vi "Trabalho2.vi"() -> ()   [LabVIEW 2009]
uses:
  <vilib>/NXT/Block Support/NXT_InputPort.ctl
  <vilib>/NXT/Block Support/NXT_ButtonSelector.ctl
  <vilib>/NXT/Subs/MotorOutput.ctl
  <vilib>/NXT/Dual Mode Library/Waits/Wait_Num.vi
  <vilib>/NXT/Dual Mode Library/Display/drawText.vi
  <vilib>/NXT/Dual Mode Library/Sensors/Light_On.vi
  <vilib>/NXT/Dual Mode Library/Sensors/readNXTButton.vi
  <vilib>/NXT/Dual Mode Library/Sensors/Touch_Pressed.vi
  <vilib>/NXT/Dual Mode Library/Sensors/Sound_dB.vi
  <vilib>/NXT/Dual Mode Library/Sensors/Sonar_cm.vi
  <vilib>/NXT/Subs/NXT_SteeringOutputPort.ctl
panel:
  out "Verificacao":bool[](array[boolean])
  out "Cor Inicial":i16
  out "Toque\nPressionado":bool
  out "Visor":string
  out "Ruído":i16(slide) scale=0.0..100.0
  out "Luminosidade":i16
  out "Distância":i16
  out "Botao\nPressionado":bool
  # "O Mindstorms irá ficar no seguinte loop até que o botão central seja precionado:\nAciona os motores B e C para frente.\nMostrará os valores dos sensores na tela.\nCaso seja detectado: uma distância menor que 50cm, ou um ruído maior que 70dB, ou o sensor de toque seja precionado ou haja uma mudança de cor. O Mindstorms irá executar a seguinte rotina:\nIrá desligar os motores B e C.\nIrá ligar os motores B e C para trás e dará cinco voltas.\nSelecionará aleatoriamente um lado (direita/esquerda).\nEmitirá um som \"äleatório\".\nVirará 180 graus para o lado escolhido.\nE voltará ao loop."
  # "Configuração:\nOUT_A: GARRA\nOUT_B: RODA DA ESQUERDA\nOUT_C: RODA DA DIREITA\nIN_1: SENSOR DE TOQUE\nIN_2: SENSOR SONORO\nIN_3: SENSOR LUMINOSO\nIN_4: SENSOR ULTRA-SOM"
  # "1 - Distância menor que 50cm\n2 - Mudança de cor detectada\n3 - Ruído maior que 70dB\n4 - Toque precionado"
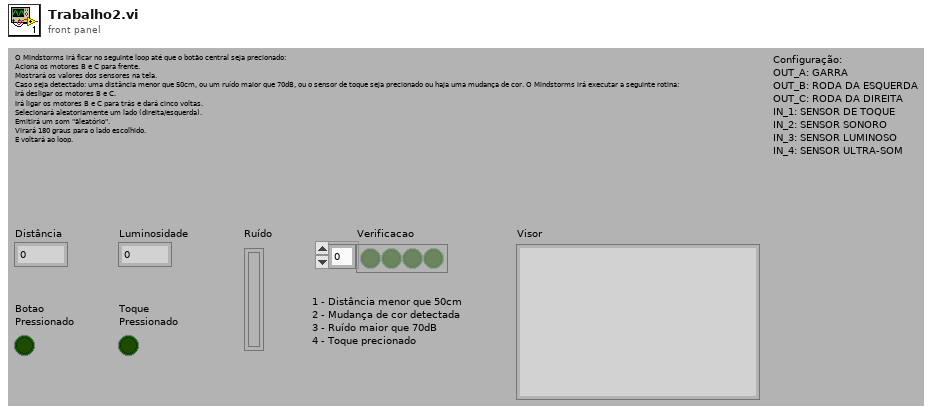
[diagram p1: front panel]
types:
  T1 = typedef "MotorOutput.ctl" = u8
  T2 = typedef "NXT_InputPort.ctl" = u8
  T3 = typedef "LVHSConnector.ctl" = cluster{"error":errorcluster, "address":string, "NXT #":i32, "Show Error":bool, "Connection":u16}
  T4 = typedef "NXT_ButtonSelector.ctl" = u16
  T5 = typedef "NXT_SteeringOutputPort.ctl" = u16
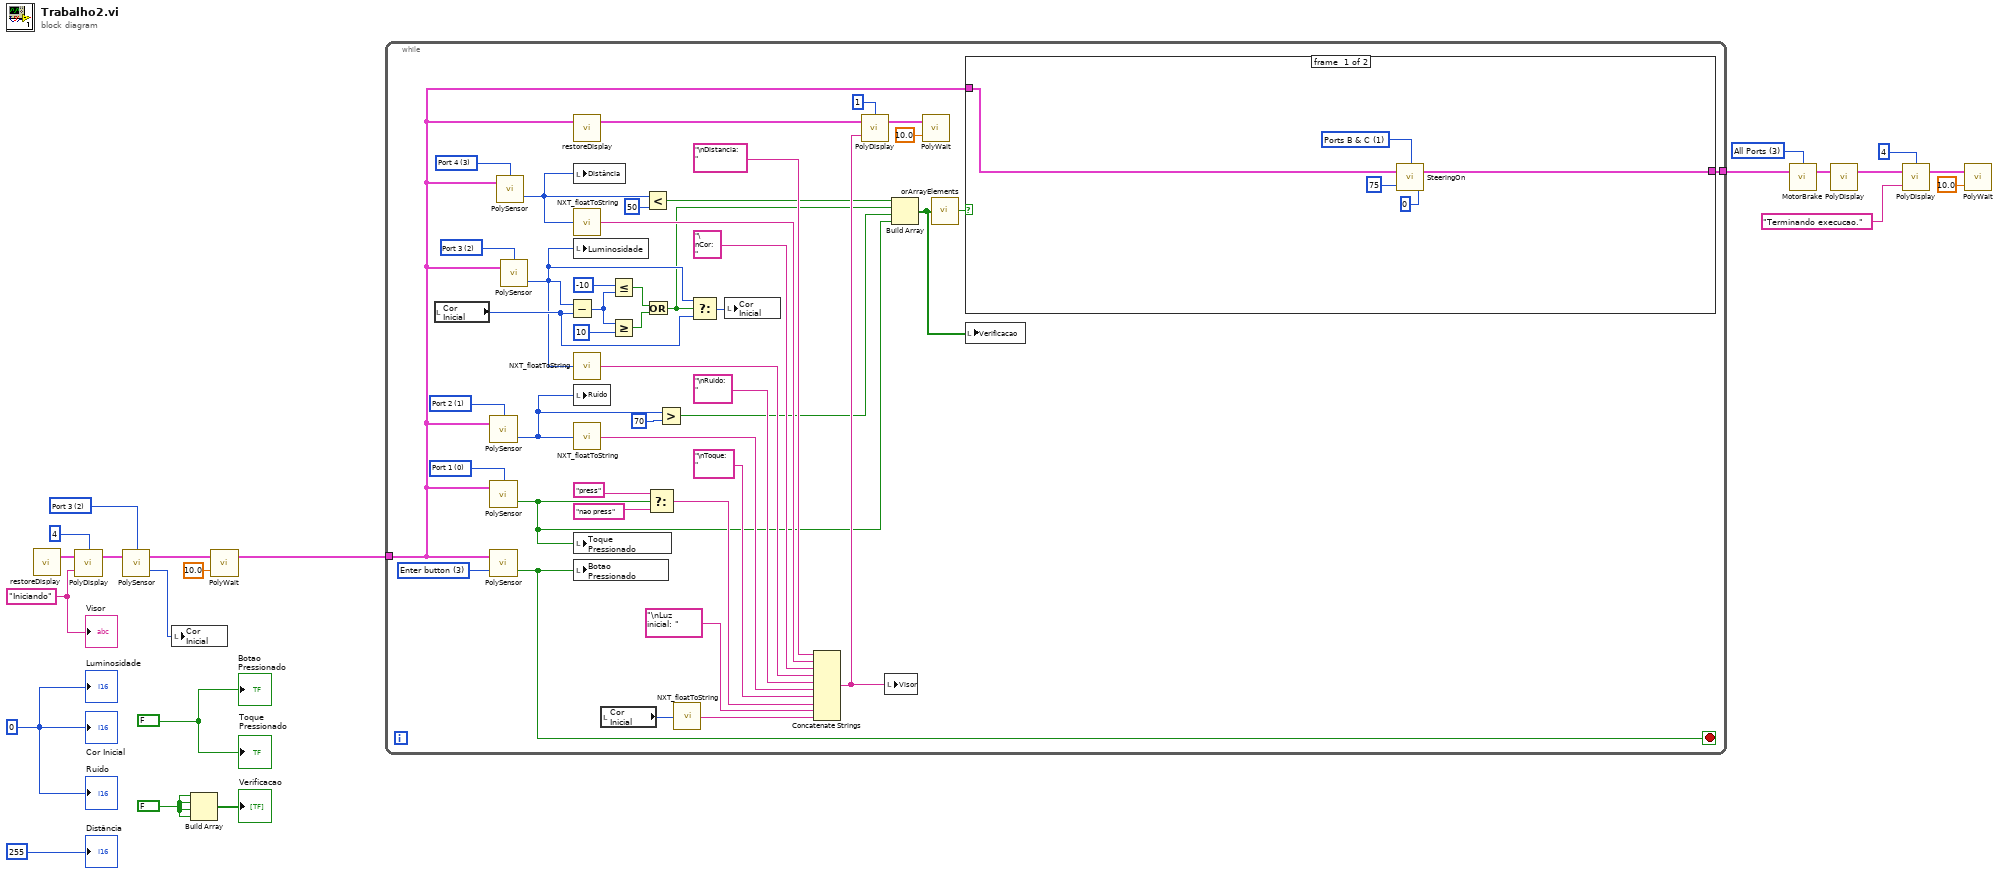
[diagram p0: block diagram]
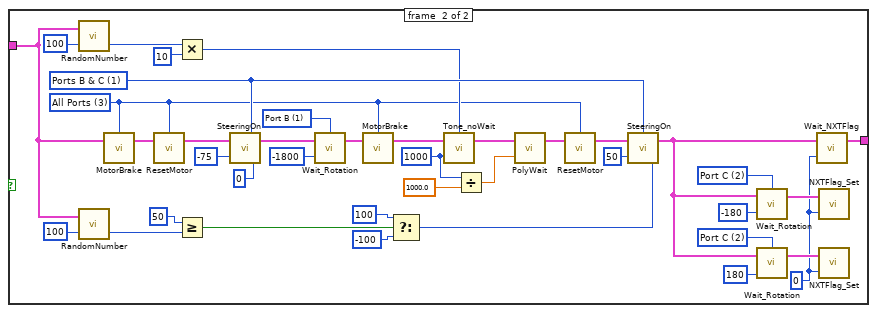
[diagram p2: hidden frame]
diagram:
  w1 = FALSE
  w14 = T1 3 items=["Port A", "Port B", "Port C", "All Ports"] ("Output Port (All Ports)")
  w10 = T2 2 items=["Port 1", "Port 2", "Port 3", "Port 4"] ("Input Port")
  w21 = "Iniciando"
  w20 = FALSE
  w4 = i16 0
  n1 = call <vilib>:"restoreDisplay.vi"() -> ("NXT"=w15:T3)  [unwired: 4 in]
  n2 = call-poly <vilib>:"PolyDisplay.vi"("Text"=w21, "NXT"=w15, "Line"=i16 4) -> ("NXT"=w6:T3)  [unwired: 1 in]
  n3 = call-poly <vilib>:"PolySensor.vi"("NXT"=w6, "Port (Port 3)"=w10) -> ("Scaled Value"=w9:i16, "NXT"=w7:T3)  [unwired: 1 in]
  n4 = local write "Cor Inicial"(w9) -> ()
  n5 = Build Array(w1, w1, w1, w1) -> (→"Verificacao":bool[])
  n6 = call-poly <vilib>:"PolyWait.vi"("Time (1 sec)"=sgl 10.0, "NXT"=w7) -> ("NXT"=w5:T3)  [unwired: 2 in]
  n7 = while {
    tunnel: w5 -> [w42]
    tunnel: [w41] -> w3
    stop <- w66 stop-if-true
    w47 = T4 3 items=["Enter button"=3, "Left button"=2, "Right button"=1] ("Button (Enter button)")
    w62 = T2 3 items=["Port 1", "Port 2", "Port 3", "Port 4"] ("Input Port")
    w63 = T2 2 items=["Port 1", "Port 2", "Port 3", "Port 4"] ("Input Port")
    w64 = T2 1 items=["Port 1", "Port 2", "Port 3", "Port 4"] ("Input Port")
    w65 = T2 0 items=["Port 1", "Port 2", "Port 3", "Port 4"] ("Input Port")
    n8 = local read "Cor Inicial"() -> (w30:i16)
    n9 = call-poly <vilib>:"PolySensor.vi"("NXT"=w42, "Port (Port 2)"=w64) -> ("Sound (dB)"=w26:i16)  [unwired: 1 in, 1 out]
    n10 = call-poly <vilib>:"PolySensor.vi"("NXT"=w42, "Port (Port 1)"=w65) -> ("Yes / No"=w24:bool)  [unwired: 1 in, 1 out]
    n11 = call-poly <vilib>:"PolySensor.vi"("Button (Enter button)"=w47, "NXT"=w42) -> ("Yes/No"=w66:bool)  [unwired: 1 in, 1 out]
    n12 = call-poly <vilib>:"PolySensor.vi"("NXT"=w42, "Port (Port 4)"=w62) -> ("Distance (cm)"=w39:i16)  [unwired: 1 in, 1 out]
    n13 = call-poly <vilib>:"PolySensor.vi"("NXT"=w42, "Port (Port 3)"=w63) -> ("Scaled Value"=w29:i16)  [unwired: 1 in, 1 out]
    n14 = Subtract(x=w29, y=w30) -> (x-y=w34:i16)
    n15 = call <vilib>:"restoreDisplay.vi"("NXT"=w42) -> ("NXT"=w46:T3)  [unwired: 3 in]
    n16 = local write "Distância"(w39) -> ()
    n17 = call <vilib>:"NXT_floatToString.vi"("number"=w39) -> ("string"=w58:string)
    n18 = local write "Luminosidade"(w29) -> ()
    n19 = call <vilib>:"NXT_floatToString.vi"("number"=w29) -> ("string"=w56:string)
    n20 = local write "Ruído"(w26) -> ()
    n21 = call <vilib>:"NXT_floatToString.vi"("number"=w26) -> ("string"=w52:string)
    n22 = local write "Toque\nPressionado"(w24) -> ()
    n23 = local write "Botao\nPressionado"(w66) -> ()
    n24 = local read "Cor Inicial"() -> (w45:i16)
    n25 = Less Or Equal?(x=i16 -10, y=w34) -> (x <= y?=w31:bool)
    n26 = Greater Or Equal?(x=w34, y=i16 10) -> (x >= y?=w32:bool)
    n27 = Less?(x=w39, y=i16 50) -> (x < y?=w37:bool)
    n28 = Or(x=w31, y=w32) -> (x .or. y?=w28:bool)
    n29 = Select(t="press", s=w24, f="nao press") -> (s? t:f=w54:string)
    n30 = Greater?(x=w26, y=i16 70) -> (0:w25:bool)
    n31 = call <vilib>:"NXT_floatToString.vi"("number"=w45) -> ("string"=w43:string)
    n32 = Select(t=w29, s=w28, f=w30) -> (s? t:f=w36:i16)
    n33 = local write "Cor Inicial"(w36) -> ()
    n34 = Concatenate Strings("\nDistancia: ", w58, "\nCor: ", w56, "\nRuido: ", w52, "\nToque: ", w54, "\nLuz inicial: ", w43) -> (w48:string)
    n35 = call-poly <vilib>:"PolyDisplay.vi"("Text"=w48, "NXT"=w46, "Line"=i16 1) -> ("NXT"=w49:T3)  [unwired: 1 in]
    n36 = local write "Visor"(w48) -> ()
    n37 = Build Array(w37, w28, w25, w24) -> (w23:bool[])
    n38 = call-poly <vilib>:"PolyWait.vi"("Time (1 sec)"=sgl 10.0, "NXT"=w49) -> ()  [unwired: 2 in, 1 out]
    n39 = call <vilib>:"orArrayElements.vi"("Boolean Array"=w23) -> ("Logical OR"=w40:bool)
    n40 = local write "Verificacao"(w23) -> ()
    n41 = case shown="True" w40 {
      tunnel: w42 -> [w68 w107]
      tunnel: [w67 w72] -> w41
      frame #0 {
        w69 = T5 1 items=["Ports A & B", "Ports B & C", "Ports A & C"] ("Output Port")
        n42 = call <vilib>:"SteeringOn.vi"("Power (75)"=75, "Steering (100)"=0, "NXT"=w68, "Output Ports"=w69) -> ("NXT"=w67:T3)
      }
      frame #1 {
        w76 = u8 1 items=["Port A", "Port B", "Port C"] ("Output Port")
        w80 = i8 0
        w87 = T1 2 items=["Port A", "Port B", "Port C", "All Ports"] ("Output Port (All Ports)")
        w86 = T1 2 items=["Port A", "Port B", "Port C", "All Ports"] ("Output Port (All Ports)")
        w91 = u16 1000
        w73 = T1 3 items=["Port A", "Port B", "Port C", "All Ports"] ("Output Port (All Ports)")
        w106 = T5 1 items=["Ports A & B", "Ports B & C", "Ports A & C"] ("Output Port")
        n43 = call <vilib>:"RandomNumber.vi"("Max Value"=i16 100, "NXT"=w107) -> ("Random Number"=w102:u16)  [unwired: 1 in, 1 out]
        n44 = call <vilib>:"RandomNumber.vi"("Max Value"=i16 100, "NXT"=w107) -> ("Random Number"=w98:u16)  [unwired: 1 in, 1 out]
        n45 = call <vilib>:"MotorBrake.vi"("NXT"=w107, "Port (All Ports)"=w73) -> ("NXT"=w79:T3)  [unwired: 2 in]
        n46 = call <vilib>:"ResetMotor.vi"("NXT"=w79, "Port (All Ports)"=w73) -> ("NXT"=w78:T3)  [unwired: 2 in]
        n47 = Multiply(x=w102, y=u16 10) -> (x*y=w100:u16)
        n48 = Greater Or Equal?(x=u16 50, y=w98) -> (x >= y?=w97:bool)
        n49 = call <vilib>:"SteeringOn.vi"("Power (75)"=-75, "Steering (100)"=0, "NXT"=w78, "Output Ports"=w106) -> ("NXT"=w77:T3)
        n50 = call <vilib>:"Wait_Rotation.vi"("Position Change (180)"=-1800, "NXT"=w77, "Port (Port A)"=w76) -> ("NXT"=w88:T3)  [unwired: 1 in]
        n51 = call <vilib>:"MotorBrake.vi"("NXT"=w88, "Port (All Ports)"=w73) -> ("NXT"=w90:T3)  [unwired: 2 in]
        n52 = Select(t=100, s=w97, f=-100) -> (s? t:f=w99:i32)
        n53 = call <vilib>:"Tone_noWait.vi"("Duration (500 ms)"=w91, "NXT"=w90, "Tone (440 Hz)"=w100) -> ("NXT"=w104:T3)  [unwired: 1 in]
        n54 = Divide(x=w91, y=sgl 1000.0) -> (x/y=w93:sgl)
        n55 = call-poly <vilib>:"PolyWait.vi"("Time (1 sec)"=w93, "NXT"=w104) -> ("NXT"=w75:T3)  [unwired: 2 in]
        n56 = call <vilib>:"ResetMotor.vi"("NXT"=w75, "Port (All Ports)"=w73) -> ("NXT"=w74:T3)  [unwired: 2 in]
        n57 = call <vilib>:"SteeringOn.vi"("Power (75)"=50, "Steering (100)"=w99, "NXT"=w74, "Output Ports"=w106) -> ("NXT"=w81:T3)
        n58 = call <vilib>:"Wait_Rotation.vi"("Position Change (180)"=-180, "NXT"=w81, "Port (Port A)"=w86) -> ("NXT"=w82:T3)  [unwired: 1 in]
        n59 = call <vilib>:"Wait_Rotation.vi"("Position Change (180)"=180, "NXT"=w81, "Port (Port A)"=w87) -> ("NXT"=w83:T3)  [unwired: 1 in]
        n60 = call <vilib>:"Wait_NXTFlag.vi"("NXT Flag Number"=w80, "NXT"=w81) -> ("NXT"=w72:T3)  [unwired: 2 in]
        n61 = call <vilib>:"NXTFlag_Set.vi"("NXT Flag Number"=w80, "NXT"=w82) -> ()  [unwired: 2 in, 1 out]
        n62 = call <vilib>:"NXTFlag_Set.vi"("NXT Flag Number"=w80, "NXT"=w83) -> ()  [unwired: 2 in, 1 out]
      }
    }
  }
  n63 = call <vilib>:"MotorBrake.vi"("NXT"=w3, "Port (All Ports)"=w14) -> ("NXT"=w12:T3)  [unwired: 2 in]
  n64 = call-poly <vilib>:"PolyDisplay.vi"("NXT"=w12) -> ("NXT"=w18:T3)  [unwired: 3 in]
  n65 = call-poly <vilib>:"PolyDisplay.vi"("Text"="Terminando execucao.", "NXT"=w18, "Line"=i16 4) -> ("NXT"=w11:T3)  [unwired: 1 in]
  n66 = call-poly <vilib>:"PolyWait.vi"("Time (1 sec)"=sgl 10.0, "NXT"=w11) -> ()  [unwired: 2 in, 1 out]
  "Botao\nPressionado" <- w20
  "Distância" <- i16 255
  "Luminosidade" <- w4
  "Ruído" <- w4
  "Visor" <- w21
  "Toque\nPressionado" <- w20
  "Cor Inicial" <- w4
